vi "NumericText.vi"(8 "error in":errorcluster, 11 "GObj Refnum":refnum<vi>) -> (0 "error out":errorcluster, 3 "Numeric Text out":refnum<class "NumericText.lvclass">)   [LabVIEW 2014, in "NumericText.lvclass"]
uses:
  NumericText.lvclass
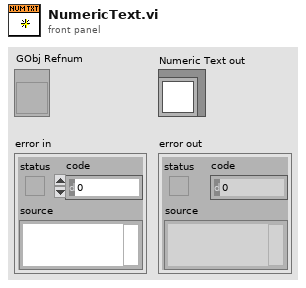
[diagram p1: front panel]
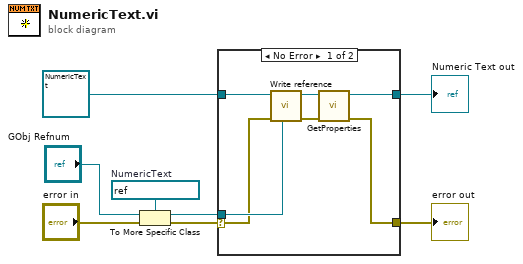
[diagram p0: block diagram]
diagram:
  w6 = refnum<vi> refnum  # NumericText
  n1 = To More Specific Class(target class=w6, reference="GObj Refnum", error in="error in") -> (specific class reference=w3:refnum<vi>, error out=w4:errorcluster)
  n2 = case shown="No Error" w4 {
    selector: w4 -> [w12 w17]
    tunnel: refnum<class "NumericText.lvclass"> refnum ("Text in") -> [w15 w16]
    tunnel: w3 -> [w13 _]
    tunnel: [w10 w16] -> w1
    tunnel: [w9 w17] -> w2
    frame No Error {
      n3 = call-dynamic "Write reference.vi"("reference"=w13, "error in"=w12, "GObject in"=w15) -> ("error out"=w11:errorcluster, "GObject out"=w14:refnum<class "NumericText.lvclass">)  [unwired: 5 in]
      n4 = call-dynamic "GetProperties.vi"("error in"=w11, "Numeric Text in"=w14) -> ("error out"=w9:errorcluster, "Numeric Text out"=w10:refnum<class "NumericText.lvclass">)  [unwired: 8 in]
    }
    frame Error {
    }
  }
  "error out" <- w2
  "Numeric Text out" <- w1
